vi "Introspection Core.vi"(8 "error in (no error)":errorcluster, 11 "KIT-QVA in":refnum<class "KIT-QVA.lvclass">) -> (0 "error out":errorcluster, 2 "CS++Messages":refnum<class "Message.lvclass">[](array[class]), 3 "KIT-QVA out":refnum<class "KIT-QVA.lvclass">)   [LabVIEW 2014, in "KIT-QVA.lvlib" / "KIT-QVA.lvclass"]
doc: "This vi delivers a list with all messages this actor reacts to. \n\nNote that all inherited classes have to overwrite it."
uses:
  KIT-QVA.lvclass
  <vilib>/ActorFramework/Message/Message.lvclass
  KIT-QVA Messages/Quench Msg/Quench Msg.lvclass
  KIT-QVA Messages/Mute Single Msg/Mute Single Msg.lvclass
  KIT-QVA Messages/Mute All Msg/Mute All Msg.lvclass
  KIT-QVA Messages/Control Mode Msg/Control Mode Msg.lvclass
  KIT-QVA Messages/Auto Mute Msg/Auto Mute Msg.lvclass
  KIT-QVA Messages/Acknowledge Fault Msg/Acknowledge Fault Msg.lvclass
  CSPP_Core/Actors/CS++DeviceActor/CS++DeviceActor.lvclass
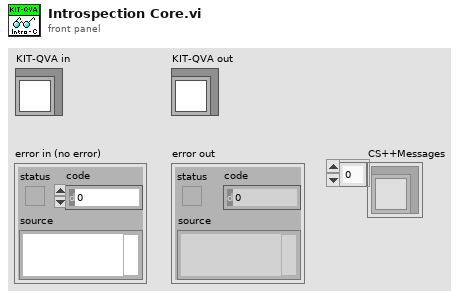
[diagram p1: front panel]
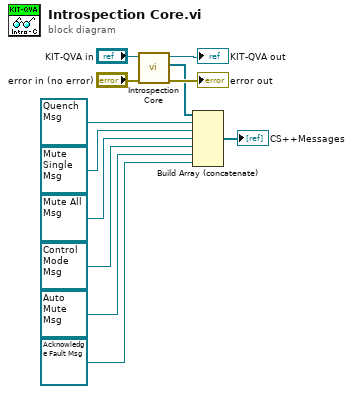
[diagram p0: block diagram]
diagram:
  n1 = call-parent "Introspection Core.vi"("error in (no error)"="error in (no error)", "CS++DeviceActor in"="KIT-QVA in") -> ("error out"=→"error out":errorcluster, "CS++Messages"=w11:refnum<class "Message.lvclass">[], "CS++DeviceActor out"=→"KIT-QVA out":refnum<class "KIT-QVA.lvclass">)  [unwired: 7 in]
  n2 = Build Array (concatenate)(w11, refnum<class "Quench Msg.lvclass"> refnum ("KIT-QVA.lvlib:Quench Msg.lvclass"), refnum<class "Mute Single Msg.lvclass"> refnum ("KIT-QVA.lvlib:Mute Single Msg.lvclass"), refnum<class "Mute All Msg.lvclass"> refnum ("KIT-QVA.lvlib:Mute All Msg.lvclass"), refnum<class "Control Mode Msg.lvclass"> refnum ("KIT-QVA.lvlib:Control Mode Msg.lvclass"), refnum<class "Auto Mute Msg.lvclass"> refnum ("KIT-QVA.lvlib:Auto Mute Msg.lvclass"), refnum<class "Acknowledge Fault Msg.lvclass"> refnum ("KIT-QVA.lvlib:Acknowledge Fault Msg.lvclass")) -> (→"CS++Messages":refnum<class "Message.lvclass">[])
